vi "Part 2.vi"(11 "Input":string) -> (3 "Output":i64)   [LabVIEW 2021]
uses:
  490f0501-92ba-4882-bc2c-926fe380afa5.vi
  <userlib>/_OpenG.lib/string/string.llb/Convert EOLs (String)__ogtk.vi
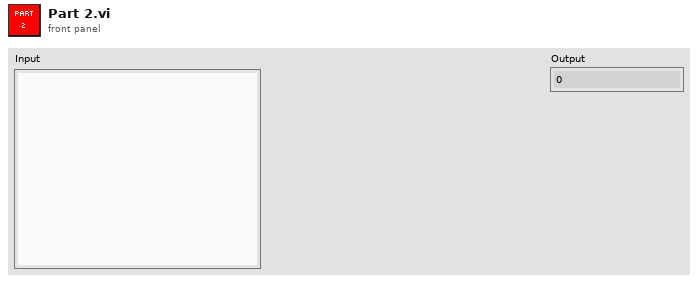
[diagram p1: front panel]
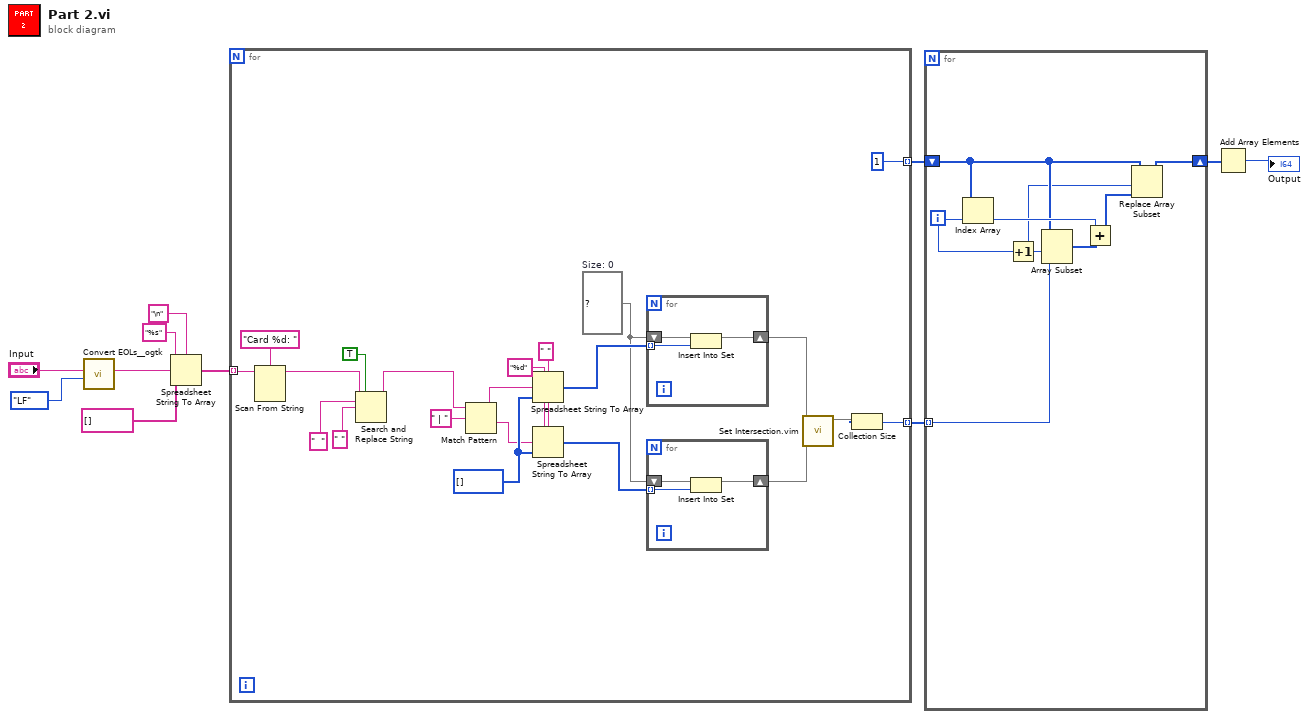
[diagram p0: block diagram]
diagram:
  n1 = call-poly <userlib>:"Convert EOLs__ogtk.vi"("Convert to:"=enum16{"CR", "LF", "CRLF"}."LF", "String in"="Input") -> ("String out"=w7:string)  [unwired: 9 in]
  n2 = Spreadsheet String To Array(delimiter (Tab)="\n", format string="%s", spreadsheet string=w7, array type (2D Dbl)=string[] []) -> (array=w5:string[])
  n3 = for {
    tunnel: w5 -> [w32] mode=indexing
    tunnel: [w13] -> w4 mode=indexing
    tunnel: [i64 1] -> w3 mode=indexing
    w18 = set{i64} {}  # Size: 0
    w25 = " "
    w26 = "%d"
    w29 = i64[] []
    n4 = Scan From String(format string="Card %d: ", input string=w32) -> (remaining string=w24:string)  [unwired: 4 in, 2 out]
    n5 = Search and Replace String(replace all?=TRUE, input string=w24, search string="  ", replace string=" ") -> (result string=w23:string)  [unwired: 4 in, 3 out]
    n6 = Match Pattern(string=w23, regular expression=" | ") -> (before substring=w27:string, after substring=w28:string)  [unwired: 1 in, 2 out]
    n7 = Spreadsheet String To Array(delimiter (Tab)=w25, format string=w26, spreadsheet string=w27, array type (2D Dbl)=w29) -> (array=w19:i64[])
    n8 = Spreadsheet String To Array(delimiter (Tab)=w25, format string=w26, spreadsheet string=w28, array type (2D Dbl)=w29) -> (array=w17:i64[])
    n9 = for {
      tunnel: w19 -> [w38] mode=indexing
      shift-right: [w37] -> w15
      shift-left: w18 -> [w36]
      n10 = Insert Into Set(10:w38, 11:w36) -> (3:w37:set{i64})  [unwired: 1 out]
    }
    n11 = for {
      tunnel: w17 -> [w35] mode=indexing
      shift-right: [w34] -> w16
      shift-left: w18 -> [w33]
      n12 = Insert Into Set(10:w35, 11:w33) -> (3:w34:set{i64})  [unwired: 1 out]
    }
    n13 = call "Set Intersection.vim"("set 2"=w16, "set 1"=w15) -> ("intersection"=w14:set{i64})  [unwired: 9 in]
    n14 = Collection Size(1:w14) -> (0:w13:i32)
  }
  n15 = for {
    tunnel: w4 -> [w44] mode=indexing
    shift-right: [w39] -> w2
    shift-left: w3 -> [w42]
    i -> [w46]
    n16 = Index Array(array=w42, index=w46) -> (element=w45:i64)
    n17 = Increment(x=w46) -> (x+1=w40:i32)
    n18 = Array Subset(array=w42, index=w40, length=w44) -> (w43:i64[])
    n19 = Add(x=w45, y=w43) -> (x+y=w41:i64[])
    n20 = Replace Array Subset(array=w42, new element=w41, index=w40) -> (w39:i64[])
  }
  n21 = Add Array Elements(numeric array=w2) -> (sum=→"Output":i64)
